vi "Error Strings Global Internal.vi"() -> ()   [LabVIEW 2020]
panel:
  out "5071":string="Latched booleans are not supported for measurement parameters. Change the mechanical action on these controls:\n%s"
  out "5070":string="The following enums contain at least one item with an invalid character. Enum strings must not contain the \";\" or \"=\" characters.\n\n%s"
  out "5069":string="Expected a single session. Found %d sessions."
  out "5068":string="The pin or relay name(s) input is not valid. When specifying a single pin, the name must be non-empty. When specifying multiple pins, the array must have at least one name and every name must be non-empty."
  out "5067":string="No connections match for %s %s."
  out "5066":string="Could not start the measurement because the discovery service is not installed. Install InstrumentStudio and try again."
  out "5065":string="Attempted to use session reservation that has been unreserved."
  out "5064":string="No connections match pin or relay name(s) '%s' with the specified criteria: %s"
  out "5063":string="No connections match the specified criteria: %s"
  out "5062":string="Expected a single connection. Found %d connections."
  out "5061":string="Found zero sessions to create."
  out "5060":string="The IInstrument provided an empty Instrument Type ID. Creating sessions requires a valid Instrument Type ID."
  out "5059":string="Attempted to create session for \"%s\" but session already exists."
  out "5058":string="Expected to create exactly 1 session but found %d sessions."
  out "5057":string="Invalid measurement metadata. The following parameter names in `Get Type Specializations.vi` do not match any controls in `Measurement Configuration.ctl` or indicators in `Measurement Results.ctl`:"
  out "5056":string="Timed out waiting for discovery service to start."
  out "5055":string="Failed to read the discovery service key file."
  out "5054":string="Failed to get the discovery service key file size."
  out "5053":string="Failed to read the discovery service key file.\nEnsure that the discovery service is running."
  out "5052":string="The %s driver is not installed."
  out "5051":string="<Unused Error>"
  out "5050":string="<b>Invalid Data Types</b>\n\nInvalid measurement configurations:\n%s\n\nInvalid measurement results:\n%s\n\nThe data type of these controls or indicators are not supported by the Measurement Service. For arrays, enums, and rings, the underlying representation must be a supported data type.\n\nSee \"https://www.ni.com/r/measurementlinkdatatypes\" for details."
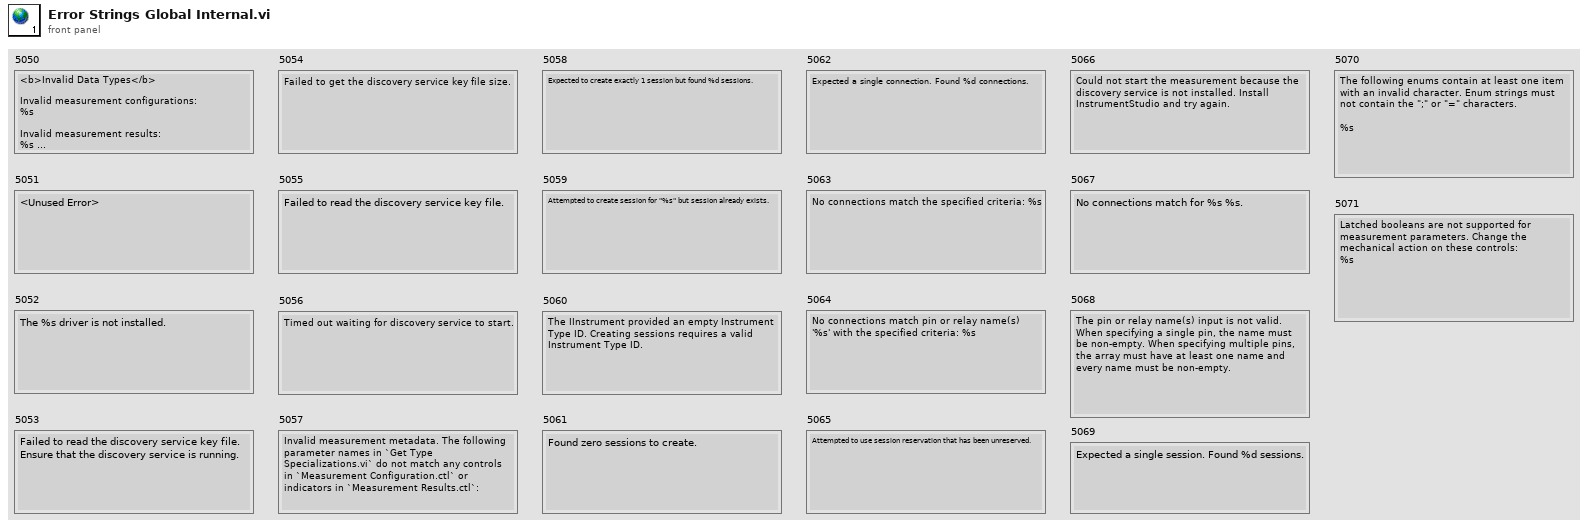
[diagram p1: front panel]
diagram:
